vi "Read X column ref.vi"(8 "error in (no error)":errorcluster, 11 "XY WFRM Plot in":refnum<class "XY WFRM Plot.lvclass">) -> (0 "error out":errorcluster, 2 "X column ref":refnum<vi>, 3 "XY WFRM Plot out":refnum<class "XY WFRM Plot.lvclass">)   [LabVIEW 2015, in "XY WFRM Plot.lvclass"]
uses:
  XY WFRM Plot.lvclass
  XY WFRM Plot.lvclass/XY WFRM Plot.ctl
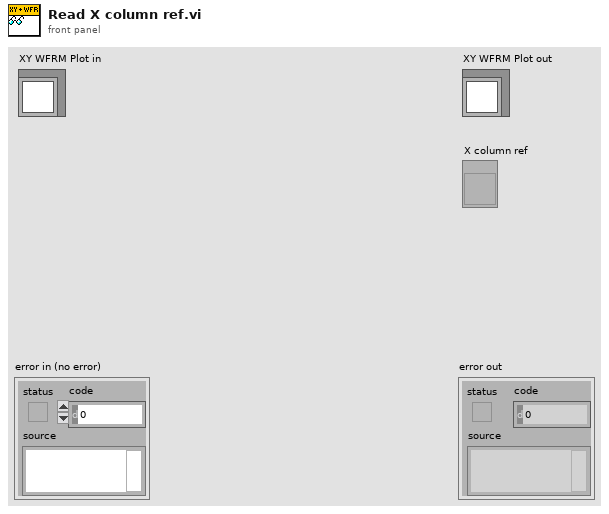
[diagram p1: front panel]
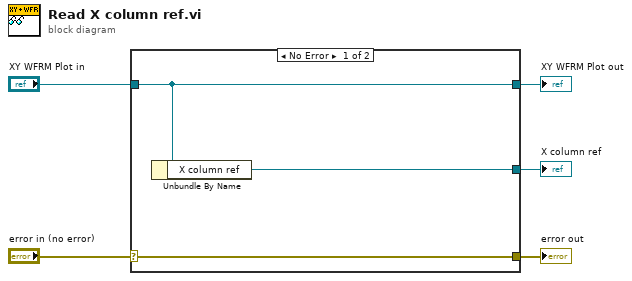
[diagram p0: block diagram]
diagram:
  n1 = case shown="No Error" "error in (no error)" {
    selector: "error in (no error)" -> [w8 w9]
    tunnel: [w8 w9] -> w4
    tunnel: [w7 w10] -> w2
    tunnel: "XY WFRM Plot in" -> [w7 w10]
    tunnel: [w6 _] -> w1
    frame No Error {
      n2 = Unbundle By Name(w7) -> ("X column ref"=w6:refnum<vi>)
    }
    frame Error {
    }
  }
  "error out" <- w4
  "XY WFRM Plot out" <- w2
  "X column ref" <- w1
